vi "CRYUpdate Main Menu Recent.vi"(11 "menu tag":string) -> ()   [LabVIEW 2013]
uses:
  SubVI/CRYMain Sub Window Global.vi
  CRYMainGlobal.vi
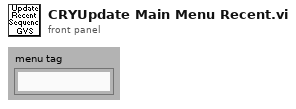
[diagram p1: front panel]
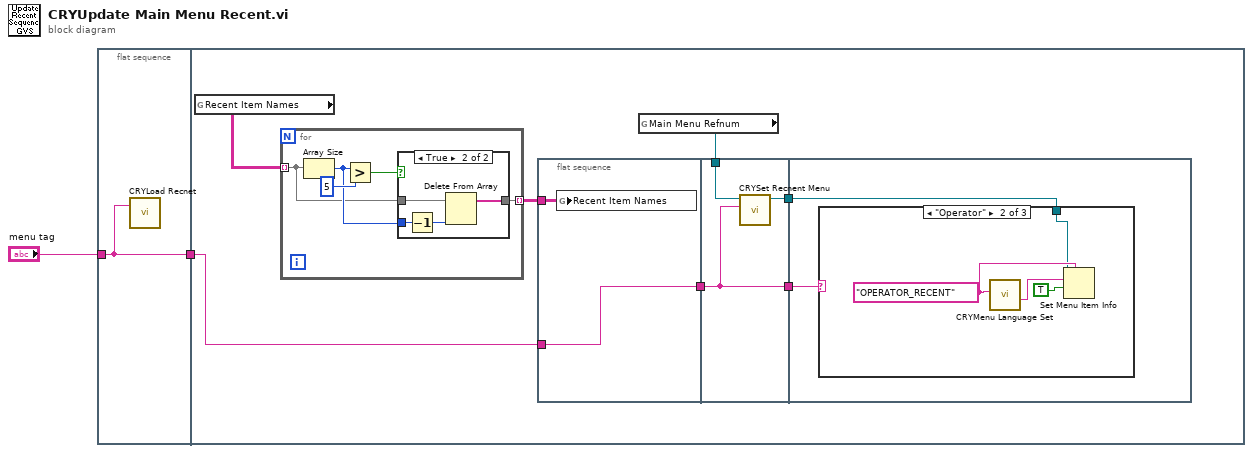
[diagram p0: block diagram]
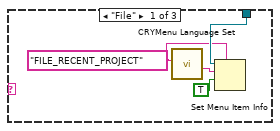
[diagram p3: hidden frame]
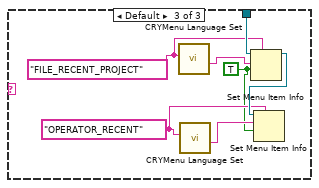
[diagram p4: hidden frame]
diagram:
  n1 = flat-sequence {
    tunnel: [w3] -> w2
    tunnel: "menu tag" -> [w3]
    tunnel: w2 -> [w6]
    frame #0 {
      n2 = call "CRYLoad Recnet.vi"("menu tag"=w3) -> ()  [unwired: 1 in, 1 out]
    }
    frame #1 {
      n3 = global read "CRYMainGlobal.vi" "Recent Item Names"() -> (w8:string[][])
      n4 = for {
        tunnel: [w15] -> w10 mode=indexing
        tunnel: w8 -> [w11] mode=indexing
        n5 = Array Size(array=w11) -> (size(s)=w13:i32)
        n6 = Greater?(x=w13, y=5) -> (0:w12:bool)
        n7 = case shown="True" w12 {
          tunnel: w11 -> [w16 w20]
          tunnel: w13 -> [_ w19]
          tunnel: [w16 w17] -> w15
          frame False {
          }
          frame True {
            n8 = Decrement(x=w19) -> (x-1=w18:i32)
            n9 = Delete From Array(array=w20, index=w18) -> (array with subset deleted=w17:string[])  [unwired: 1 in, 1 out]
          }
        }
      }
      n10 = flat-sequence {
        tunnel: w10 -> [w22]
        tunnel: w6 -> [w21]
        tunnel: [w21] -> w4
        tunnel: w9 -> [w25]
        tunnel: [w24] -> w7
        tunnel: [w23] -> w5
        tunnel: w4 -> [w23]
        tunnel: w7 -> [w27]
        tunnel: w5 -> [w26]
        frame #0 {
          n11 = global write "CRYMainGlobal.vi" "Recent Item Names"(w22) -> ()
        }
        frame #1 {
          n12 = call "CRYSet Recnent Menu.vi"("menuc tag"=w23, "Main Menu Refnum in"=w25) -> ("Main Menu Refnum out"=w24:refnum<k9>)  [unwired: 9 out]
        }
        frame #2 {
          n13 = case shown="\"Operator\"" w26 {
            tunnel: w27 -> [w30 w32 w41]
            frame "File" {
              w29 = "FILE_RECENT_PROJECT" ("menu tag")
              n14 = call "CRYMenu Language Set.vi"("sID"=w29) -> ("sMultibyte_Out"=w31:string)  [unwired: 7 in, 3 out]
              n15 = Set Menu Item Info(7:w29, 9:TRUE ("enabled"), 10:w31, 11:w30) -> ()  [unwired: 1 in, 4 out]
            }
            frame "Operator" {
              w35 = "OPERATOR_RECENT" ("menu tag")
              n16 = call "CRYMenu Language Set.vi"("sID"=w35) -> ("sMultibyte_Out"=w34:string)  [unwired: 7 in, 3 out]
              n17 = Set Menu Item Info(7:w35, 9:TRUE ("enabled"), 10:w34, 11:w32) -> ()  [unwired: 1 in, 4 out]
            }
            frame Default {
              w38 = "OPERATOR_RECENT" ("menu tag")
              w36 = TRUE ("enabled")
              w40 = "FILE_RECENT_PROJECT" ("menu tag")
              n18 = call "CRYMenu Language Set.vi"("sID"=w40) -> ("sMultibyte_Out"=w42:string)  [unwired: 7 in, 3 out]
              n19 = call "CRYMenu Language Set.vi"("sID"=w38) -> ("sMultibyte_Out"=w37:string)  [unwired: 7 in, 3 out]
              n20 = Set Menu Item Info(7:w40, 9:w36, 10:w42, 11:w41) -> (3:w39:refnum<k9>)  [unwired: 1 in, 3 out]
              n21 = Set Menu Item Info(7:w38, 9:w36, 10:w37, 11:w39) -> ()  [unwired: 1 in, 4 out]
            }
          }
        }
      }
      n22 = global read "CRYMain Sub Window Global.vi" "Main Menu Refnum"() -> (w9:refnum<k9>)
    }
  }
